vi "Collector Button Status.vi"(8 "error in":errorcluster) -> (0 "error out":errorcluster, 2 "Collect":bool, 3 "Eject":bool)   [LabVIEW 2015]
uses:
  Support/Global Objects.vi
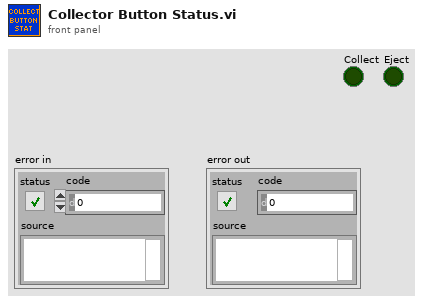
[diagram p1: front panel]
types:
  T1 = typedef "Teleop Commands.ctl" = cluster{"Throttle":dbl, "Turn":dbl, "Up Shift Commanded":bool, "Down Shift Commanded":bool, "Collect":bool, "Eject":bool, "Flywheel":bool}
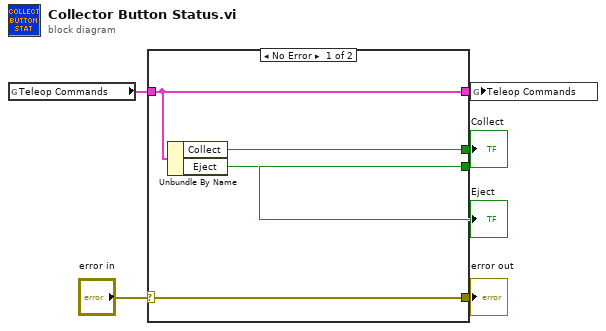
[diagram p0: block diagram]
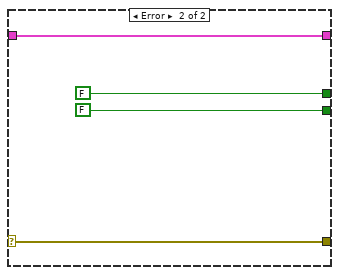
[diagram p2: hidden frame]
diagram:
  n1 = global read "Global Objects.vi" "Teleop Commands"() -> (w4:T1)
  n2 = case shown="No Error" "error in" {
    selector: "error in" -> [w10 w14]
    tunnel: [w10 w14] -> w5
    tunnel: [w9 w13] -> w3
    tunnel: w4 -> [w9 w13]
    tunnel: [w8 FALSE ("Collect")] -> w2
    tunnel: [w7 FALSE ("Eject")] -> w1
    frame No Error {
      n3 = Unbundle By Name(w9) -> ("Collect"=w8:bool, "Eject"=w7:bool)
    }
    frame Error {
    }
  }
  "error out" <- w5
  "Collect" <- w2
  "Eject" <- w1
  n4 = global write "Global Objects.vi" "Teleop Commands"(w3) -> ()
